vi "Read issue body.vi"(11 "MyComics.org_class in":refnum<class "MyComics.org_class.lvclass">) -> (2 "issue body":string, 3 "MyComics.org_class out":refnum<class "MyComics.org_class.lvclass">)   [LabVIEW 2024, in "MyComics.org_class.lvclass"]
uses:
  MyComics.org_class.lvclass
  MyComics.org_class.lvclass/MyComics.org_class.ctl
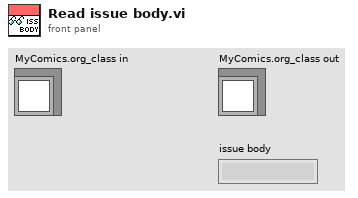
[diagram p1: front panel]
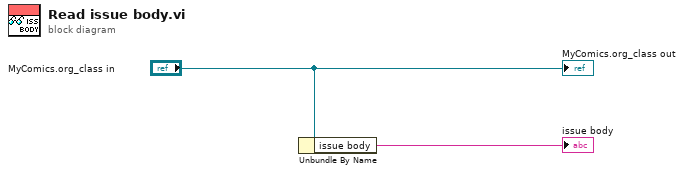
[diagram p0: block diagram]
diagram:
  n1 = Unbundle By Name("MyComics.org_class in") -> ("issue body"=→"issue body":string)
  "MyComics.org_class out" <- "MyComics.org_class in"
